vi "State_Machine.vi"(8 "error in (no error)":errorcluster caption="entrée d'erreur (pas d'erreur)", 11 "Flash_Jlink en entrée":refnum<class "P2265_SwitchOn_Test.lvclass">) -> (0 "error out":errorcluster caption="sortie d'erreur", 2 "Json_String":string, 3 "Flash_Jlink en sortie":refnum<class "P2265_SwitchOn_Test.lvclass">)   [LabVIEW 2020, in "Library Test.lvlib" / "P2265_SwitchOn_Test.lvclass"]
uses:
  P2265_SwitchOn_Test.lvclass
  C:/Users/ngarcin/OneDrive - Altyor/Standard TB/Class/Test/Test (Default)/Test (Default).lvclass
  Process/Process (Default)/Process (Default).lvclass
  Commun VI/TypeDef/Commande Relay_Board/Data_Write_Relay_Board.ctl
  <vilib>/Platform/TimedLoop/XDataNode/timing_clust.ctl
  <vilib>/Platform/TimedLoop/XDataNode/nitl_modes.ctl
  <vilib>/Platform/TimedLoop/XDataNode/wakeup.ctl
  47468121-72c4-45b5-882e-1ed00f6503c4.vi
  JSON API/Variant JSON/Variant to JSON.vi
  JSON API/JSON Value/Get Item by name array.vi
  <vilib>/Platform/TimedLoop/XDataNode/XDataNode.xnode
  Instrument/Instrument (Default)/Class Instrument (Default).lvclass
  JSON API/JSON Value/JSON Value.lvclass
  P2265_SwitchOn_Test.lvclass/P2265_SwitchOn_Test.ctl
  <vilib>/Platform/TimedLoop/XDataNode/XDNodeRunTimeDep.lvlib
  JSON API/Get Polymorphic/JSON GetSet.lvlib
  JSON API/Variant JSON/Variant JSON.lvlib
  Commun VI/Library Commun.lvlib
panel:
  out "String In progress":string
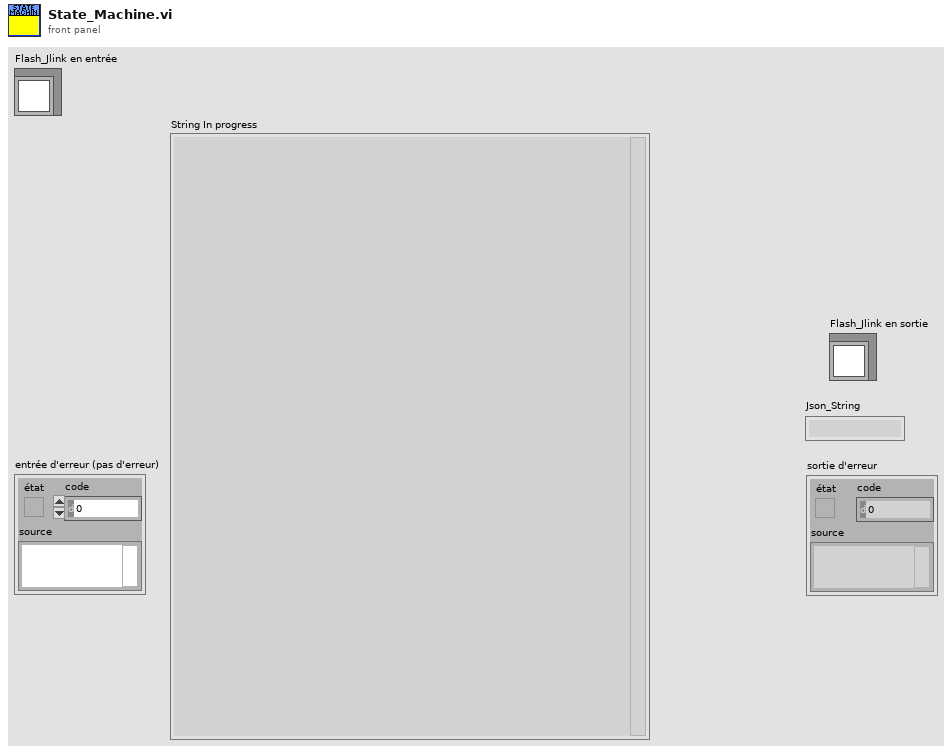
[diagram p1: front panel]
types:
  T1 = typedef "Library Commun.lvlib/Data_Write_Relay_Board.ctl" = enum16{"Enable Relays", "Disable Relays"}
  T2 = typedef "XDNodeRunTimeDep.lvlib/timing_clust.ctl" = cluster{"Expected End [f-1]":u64, "Actual End [f-1]":u64, "Finished Late? [f-1]":bool, "Expected End [i-1]":u64, "Actual End [i-1]":u64, "Finished Late? [i-1]":bool, "Expected Start [i]":u64, "Actual Start [i]":u64, "Expected Start [f]":u64, "Actual Start [f]":u64, "Source Name":string, "Structure Name":string, "Period":i64, "Deadline":i64, "Offset":i64, "Start":i64, "Priority":i32, "Timeout":i32, "Mode":T3, "Wakeup Reason":T4, "Error":errorcluster, "Source Type":string, "Secondary Source Type":string, "Global End Time":u64, "Global Start Time":u64, "Frame Duration":u64, "Iteration Duration":u64, "Assigned CPU":i32, "I/O Scan Engine Mode":u32}
  T3 = typedef "XDNodeRunTimeDep.lvlib/nitl_modes.ctl" = enum32{"No Change", "Process missed periods, maintain original phase", "Discard missed periods, maintain original phase", "Process missed periods, ignore original phase", "Discard missed periods, ignore original phase"}
  T4 = typedef "XDNodeRunTimeDep.lvlib/wakeup.ctl" = enum32{"Normal", "Aborted", "Asynchronous wakeup", "Timing source error", "Timed loop error", "Timeout"}
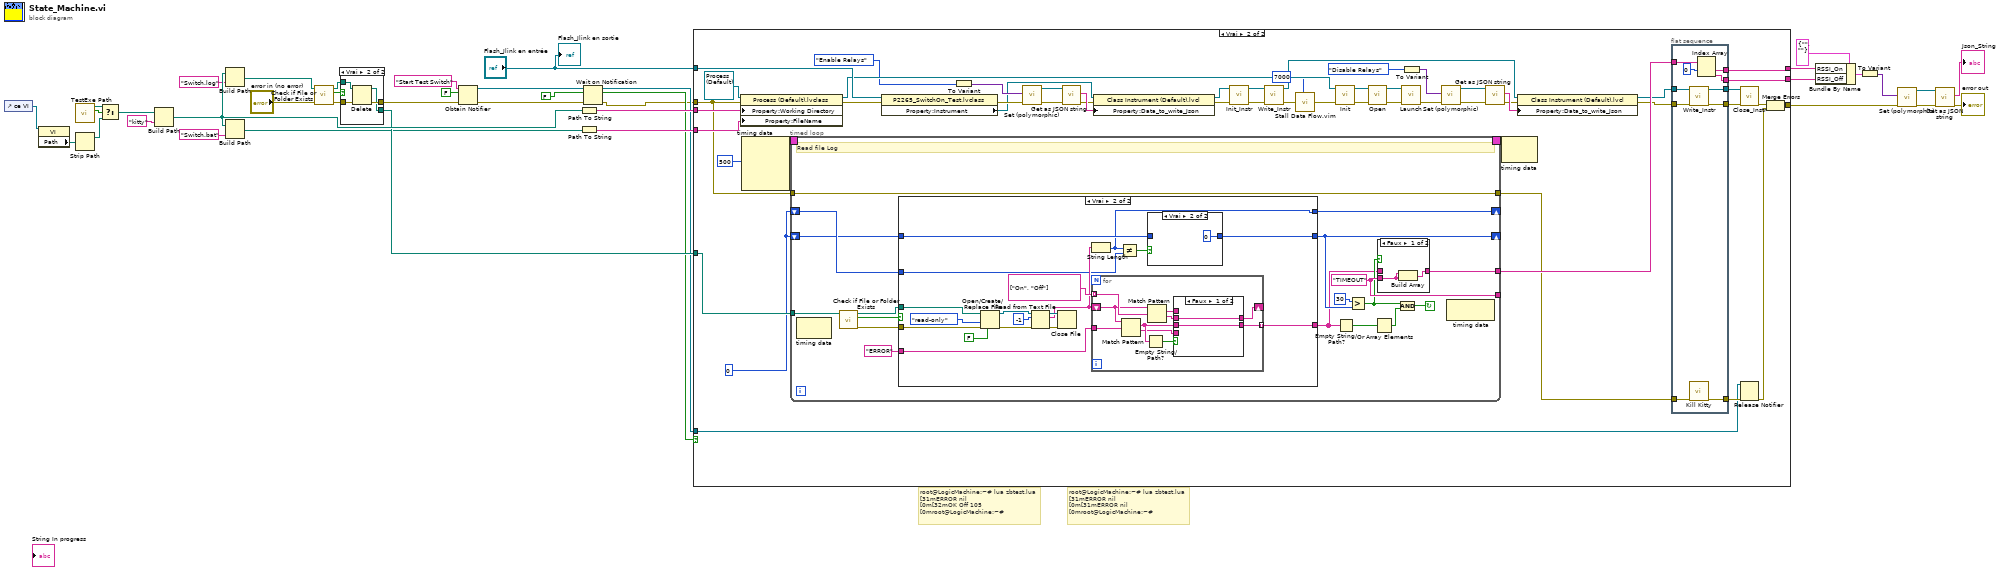
[diagram p0: block diagram]
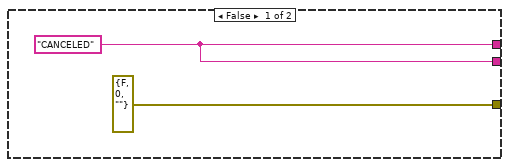
[diagram p2: hidden frame]
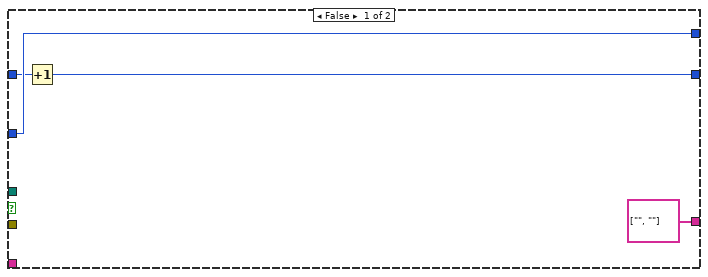
[diagram p4: hidden frame]
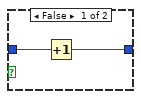
[diagram p5: hidden frame]
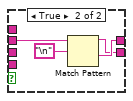
[diagram p6: hidden frame]
diagram:
  # "root@LogicMachine:~# lua zbtest.lua\n[31mERROR\tnil\n[0m[32mOK\tOff\t105\n[0mroot@LogicMachine:~#"
  # "root@LogicMachine:~# lua zbtest.lua\n[31mERROR\tnil\n[0m[31mERROR\tnil\n[0mroot@LogicMachine:~#"
  n1 = control-ref of="ce VI"() -> (w7:refnum<vi>)
  n2 = property class="VI"(reference=w7) -> ("Path"=w6:path)  [unwired: 1 in, 2 out]
  n3 = call "TestExe Path.vi"() -> ("En Exe?"=w4:bool, "Chemin Actuel"=w5:path)  [unwired: 9 in, 1 out]
  n4 = Strip Path(path=w6) -> (stripped path=w3:path)  [unwired: 1 out]
  n5 = Select(t=w5, s=w4, f=w3) -> (s? t:f=w2:path)
  n6 = Build Path(base path=w2, name or relative path="kitty" ("nom ou chemin relatif")) -> (appended path=w38:path)
  n7 = Build Path(base path=w38, name or relative path="Switch.log" ("nom ou chemin relatif")) -> (appended path=w35:path)
  n8 = Build Path(base path=w38, name or relative path="Switch.bat" ("nom ou chemin relatif")) -> (appended path=w29:path)
  n9 = call <vilib>:"Check if File or Folder Exists.vi"("error in (no error)"="error in (no error)", "path"=w35) -> ("error out"=w33:errorcluster, "file or folder exists?"=w32:bool, "dup path"=w28:path)  [unwired: 7 in]
  n10 = case shown="Vrai" w32 {
    tunnel: [w41 w45] -> w25
    tunnel: [w40 w44] -> w34
    tunnel: w28 -> [w40 w43]
    tunnel: w33 -> [w41 w42]
    frame False {
    }
    frame True {
      n11 = Delete(path (use dialog)=w43, error in=w42) -> (deleted path=w44:path, error out=w45:errorcluster)  [unwired: 3 in, 1 out]
    }
  }
  n12 = Obtain Notifier(name (unnamed)="Start Test Switch" ("nom (aucun)"), notification data type=FALSE, error in (no error)=w25) -> (notifier out=w20:refnum<notifier>, error out=w21:errorcluster)  [unwired: 1 in, 1 out]
  n13 = Path To String(path=w38) -> (string=w30:string)
  n14 = Path To String(path=w29) -> (string=w27:string)
  n15 = Wait on Notification(notifier=w20, ignore previous (F)=FALSE ("ignorer les précédents (F)"), error in (no error)=w21) -> (notifier out=w19:refnum<notifier>, notification=w18:bool, error out=w1:errorcluster)  [unwired: 1 in, 1 out]
  n16 = case shown="Vrai" w18 {
    tunnel: [errorcluster {"status"=FALSE, "code"=0, "source"=""} ("error IO") w99] -> w11
    tunnel: w34 -> [_ w98]
    tunnel: w30 -> [_ w93]
    tunnel: w27 -> [_ w91]
    tunnel: w1 -> [_ w51]
    tunnel: w19 -> [_ w83]
    tunnel: [w46 w88] -> w23
    tunnel: [w46 w87] -> w22
    tunnel: "Flash_Jlink en entrée" -> [_ w73]
    frame False {
      w46 = "CANCELED" ("expression régulière")
    }
    frame True {
      w90 = 0
      n17 = property class="Process (Default).lvclass"(reference=refnum<class "Process (Default).lvclass"> refnum ("Process (Default).lvclass"), error in=w51, "Property:Working Directory"=w93, "Property:FileName"=w91) -> (reference out=w72:refnum<class "Process (Default).lvclass">, error out=w50:errorcluster)
      n18 = node-c288(i64 500 ("Période")) -> (w82:T2)  [unwired: 3 in]
      n19 = timed-loop {
        tunnel: w98 -> [w117]
        shift-right: [w111] -> _
        shift-left: w90 -> [w110]
        shift-right: [w108] -> _
        shift-left: w90 -> [w109]
        tunnel: [w106] -> _
        tunnel: [w105] -> w89
        tunnel: [w103] -> w86
        tunnel: w51 -> [w103]
        timing: w82 -> [_]
        timing-out: [_] -> w81
        stop <- w113 continue-if-true
        w106 = "TIMEOUT" ("expression régulière")
        # "Read file Log"
        n20 = node-c288() -> ()  [unwired: 1 in, 1 out]
        n21 = call <vilib>:"Check if File or Folder Exists.vi"("path"=w117) -> ("error out"=w114:errorcluster, "file or folder exists?"=w115:bool, "dup path"=w116:path)  [unwired: 8 in]
        n22 = case shown="Vrai" w115 {
          tunnel: w116 -> [_ w142]
          tunnel: w114 -> [_ w139]
          tunnel: "ERROR" ("expression régulière") -> [_ w134]
          tunnel: [w126 w130] -> w111
          tunnel: w110 -> [w126 w129]
          tunnel: w109 -> [w125 w132]
          tunnel: [w124 w131] -> w108
          tunnel: [string[] ["", ""] w127] -> w102
          frame False {
            n23 = Increment(x=w125) -> (x+1=w124:i32)
          }
          frame True {
            n24 = Open/Create/Replace File(file path (use dialog)=w142, error in=w139, access (0:read/write)=enum16{"read/write", "read-only", "write-only"}."read-only" ("accès (0 : read/write)"), disable buffering (F)=FALSE ("désactiver la bufférisation (F)")) -> (refnum out=w141:refnum<file>, error out=w140:errorcluster)  [unwired: 2 in, 1 out]
            n25 = Read from Text File(file (use dialog)=w141, count=-1 ("nombre"), error in=w140) -> (refnum out=w137:refnum<file>, text=w133:string, error out=w138:errorcluster)  [unwired: 1 in, 1 out]
            n26 = Close File(refnum=w137, error in=w138) -> ()  [unwired: 2 out]
            n27 = String Length(string=w133) -> (length=w130:i32)
            n28 = for {
              tunnel: string[] ["On", "Off"] -> [w157] mode=indexing
              shift-right: [w150] -> _
              shift-left: w133 -> [w156]
              tunnel: w134 -> [w155]
              tunnel: [w153] -> w127 mode=indexing
              n29 = Match Pattern(string=w156, regular expression=w155) -> (match substring=w151:string, after substring=w149:string)  [unwired: 1 in, 2 out]
              n30 = Empty String/Path?(string/path=w151) -> (empty?=w154:bool)
              n31 = Match Pattern(string=w156, regular expression=w157) -> (match substring=w152:string, after substring=w148:string)  [unwired: 1 in, 2 out]
              n32 = case shown="Faux" w154 {
                tunnel: [w159 w160] -> w153
                tunnel: w152 -> [_ _]
                tunnel: w151 -> [w159 _]
                tunnel: [w158 w161] -> w150
                tunnel: w149 -> [_ _]
                tunnel: w148 -> [w158 w162]
                frame False {
                }
                frame True {
                  n33 = Match Pattern(string=w162, regular expression="\n") -> (before substring=w160:string, after substring=w161:string)  [unwired: 1 in, 2 out]
                }
              }
            }
            n34 = Not Equal?(x=w130, y=w129) -> (x != y?=w128:bool)
            n35 = case shown="Vrai" w128 {
              tunnel: w132 -> [w146 _]
              tunnel: [w145 0] -> w131
              frame False {
                n36 = Increment(x=w146) -> (x+1=w145:i32)
              }
              frame True {
              }
            }
          }
        }
        n37 = Empty String/Path?(string/path=w102) -> (empty?=w101:bool[])
        n38 = Greater?(x=30, y=w108) -> (0:w104:bool)
        n39 = Or Array Elements(Boolean array=w101) -> (logical OR=w100:bool)
        n40 = case shown="Faux" w104 {
          tunnel: w106 -> [w121 _]
          tunnel: [w120 w122] -> w105
          tunnel: w102 -> [_ w122]
          frame False {
            n41 = Build Array(w121, w121) -> (w120:string[])
          }
          frame True {
          }
        }
        n42 = Compound Arithmetic op=AND ("Opérateur arithmétique")(w104, w100) -> (w113:bool)
        n43 = node-c288() -> ()  [unwired: 1 in, 1 out]
      }
      n44 = property class="P2265_SwitchOn_Test.lvclass"(reference=w73, error in=w50) -> (error out=w74:errorcluster, "Property:Instrument"=w53:refnum<class "Class Instrument (Default).lvclass">)  [unwired: 1 out]
      n45 = To Variant(anything=Data_Write_Relay_Board."Enable Relays" ("Function")) -> (Variant=w76:variant)
      n46 = call-poly "Set (polymorphic).vi"("error in (no error)"=w74, "Variant"=w76) -> ("error out"=w78:errorcluster, "JSON Value out"=w77:refnum<class "JSON Value.lvclass">)  [unwired: 8 in]
      n47 = call "Get as JSON string.vi"("error in (no error)"=w78, "JSON Value in"=w77) -> ("error out"=w52:errorcluster, "<JSON>"=w79:string)  [unwired: 8 in]
      n48 = property class="Class Instrument (Default).lvcl"(reference=w53, error in=w52, "Property:Data_to_write_Json"=w79) -> (reference out=w54:refnum<class "Class Instrument (Default).lvclass">, error out=w55:errorcluster)
      n49 = call-dynamic "Init_Instr.vi"("error in (no error)"=w55, "Class Instrument (Default) en entrée"=w54) -> ("error out"=w62:errorcluster, "Class Instrument (Default) en sortie"=w61:refnum<class "Class Instrument (Default).lvclass">)  [unwired: 8 in]
      n50 = call-dynamic "Write_Instr.vi"("error in (no error)"=w62, "Class Multimeter (Default) en entrée"=w61) -> ("error out"=w75:errorcluster, "Class Multimeter (Default) en sortie"=w65:refnum<class "Class Instrument (Default).lvclass">)  [unwired: 8 in]
      n51 = call "Stall Data Flow.vim"("value in"=w75, "milliseconds to wait"=u32 7000) -> ("value out"=w49:errorcluster)  [unwired: 1 out]
      n52 = call-dynamic "Init.vi"("error in (no error)"=w49, "Process (Default) en entrée"=w72) -> ("error out"=w97:errorcluster, "Process (Default) en sortie"=w96:refnum<class "Process (Default).lvclass">)  [unwired: 8 in]
      n53 = call-dynamic "Open.vi"("error in (no error)"=w97, "Process (Default) en entrée"=w96) -> ("error out"=w95:errorcluster, "Process (Default) en sortie"=w94:refnum<class "Process (Default).lvclass">)  [unwired: 8 in]
      n54 = call-dynamic "Launch.vi"("error in (no error)"=w95, "Process (Default) en entrée"=w94) -> ("error out"=w67:errorcluster)  [unwired: 8 in, 1 out]
      n55 = To Variant(anything=Data_Write_Relay_Board."Disable Relays" ("Function")) -> (Variant=w66:variant)
      n56 = call-poly "Set (polymorphic).vi"("error in (no error)"=w67, "Variant"=w66) -> ("error out"=w70:errorcluster, "JSON Value out"=w69:refnum<class "JSON Value.lvclass">)  [unwired: 8 in]
      n57 = call "Get as JSON string.vi"("error in (no error)"=w70, "JSON Value in"=w69) -> ("error out"=w68:errorcluster, "<JSON>"=w71:string)  [unwired: 8 in]
      n58 = node-c288(w81) -> ()  [unwired: 1 out]
      n59 = property class="Class Instrument (Default).lvcl"(reference=w65, error in=w68, "Property:Data_to_write_Json"=w71) -> (reference out=w63:refnum<class "Class Instrument (Default).lvclass">, error out=w64:errorcluster)
      n60 = flat-sequence {
        tunnel: [w177] -> w85
        tunnel: w86 -> [w176]
        tunnel: w89 -> [w175]
        tunnel: [w174] -> w88
        tunnel: [w173] -> w87
        tunnel: w64 -> [w171]
        tunnel: w63 -> [w170]
        tunnel: [w169] -> w58
        tunnel: [w168] -> w56
        frame #0 {
          n61 = call-dynamic "Write_Instr.vi"("error in (no error)"=w171, "Class Multimeter (Default) en entrée"=w170) -> ("error out"=w169:errorcluster, "Class Multimeter (Default) en sortie"=w168:refnum<class "Class Instrument (Default).lvclass">)  [unwired: 8 in]
          n62 = call "Kill Kitty.vi"("error in (no error)"=w176) -> ("error out"=w177:errorcluster)  [unwired: 10 in]
          n63 = Index Array(array=w175, index #1=0 ("indice")) -> (element #1=w174:string, element #2=w173:string)  [unwired: 1 in]
        }
      }
      n64 = call-dynamic "Close_Instr.vi"("error in (no error)"=w58, "Class Instrument (Default) en entrée"=w56) -> ("error out"=w57:errorcluster)  [unwired: 8 in, 1 out]
      n65 = Release Notifier(notifier=w83, error in (no error)=w85) -> (error out=w84:errorcluster)  [unwired: 1 in, 2 out]
      n66 = Merge Errors(w57, w84) -> (w99:errorcluster)
    }
  }
  n67 = Bundle By Name(cluster=cluster{"RSSI_On":string, "RSSI_Off":string} {"RSSI_On"="", "RSSI_Off"=""} ("Cluster des données privées de classe"), "RSSI_On"=w23, "RSSI_Off"=w22) -> (w12:cluster{"RSSI_On":string, "RSSI_Off":string})
  n68 = To Variant(anything=w12) -> (Variant=w15:variant)
  n69 = call-poly "Set (polymorphic).vi"("error in (no error)"=w11, "Variant"=w15) -> ("error out"=w13:errorcluster, "JSON Value out"=w14:refnum<class "JSON Value.lvclass">)  [unwired: 8 in]
  n70 = call "Get as JSON string.vi"("error in (no error)"=w13, "JSON Value in"=w14) -> ("error out"=→"error out":errorcluster, "<JSON>"=→"Json_String":string)  [unwired: 8 in]
  "Flash_Jlink en sortie" <- "Flash_Jlink en entrée"
